vi "Motion Control.vi"(8 "error in (no error)":errorcluster) -> (0 "error out":errorcluster)   [LabVIEW 2020, in "Motion.lvlib"]
doc: "Message loop for handling messages pertaining to the acquisition of data from the hardware."
uses:
  Motion.lvlib
  support/PCT FGV CMD.ctl
  Acquisition State.ctl
  AM Configuration.ctl
  support/Message Queue/Message Cluster.ctl
  support/Message Queue/Enqueue Message (Single).vi
  support/Message Queue/Message Queue.lvlib
  <vilib>/ErrorRing/Error Ring.xnode
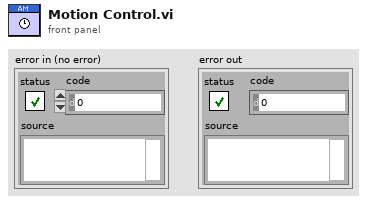
[diagram p1: front panel]
types:
  T1 = typedef "PCT FGV CMD.ctl" = enum16{"INIT", "GET", "SET"}
  T2 = typedef "Message Queue.lvlib/All Message Queues.ctl" = cluster{"UI":refnum<queue>, "Logging":refnum<queue>, "LOG":refnum<queue>, "ALARM":refnum<queue>, "Test":refnum<queue>, "Answer":refnum<queue>, "PLC":refnum<queue>, "DB":refnum<queue>, "Report":refnum<queue>, "OPC":refnum<queue>, "Procedure":refnum<queue>, "PalmSens":refnum<queue>, "SYS 7000 Reader":refnum<queue>, "SWITCH":refnum<queue>, "MOTOR":refnum<queue>, "MOTION":refnum<queue>, "HIDEN":refnum<queue>, "VALVE":refnum<queue>, "MFC":refnum<queue>, "PUMP IN":refnum<queue>, "PUMP OUT":refnum<queue>}
  T3 = typedef "PCT Data REFs.ctl" = cluster{"PLC AI Notifier":refnum<notifier>, "PS Data Queue":refnum<queue>, "BTN Queue":refnum<queue>, "PLC DI notifier":refnum<notifier>, "Timer notifier":refnum<notifier>, "DMM PS":refnum<notifier>, "DMM Gages":refnum<notifier>, "XYZ notifier":refnum<notifier>, "Test Notifier":refnum<notifier>, "Scanner notifier":refnum<notifier>, "OPC Notifier":refnum<notifier>, "HIDEN queue":refnum<queue>}
  T4 = typedef "Motion.lvlib/AM Configuration.ctl" = cluster{"Wait":dbl, "Next Step":string, "Writer Queue":refnum<queue>, "Reset":bool, "Target":dbl[]}
  T5 = typedef "Motion.lvlib/Acquisition State.ctl" = enum16{"Idle", "Initialized"}
  T6 = cluster{"Axis":enum16{"X", "Y", "Z", "A"}, "dValue":dbl}
  T7 = cluster{"Type CMD":string, "Mode CMD":string, "Main CMD":string}
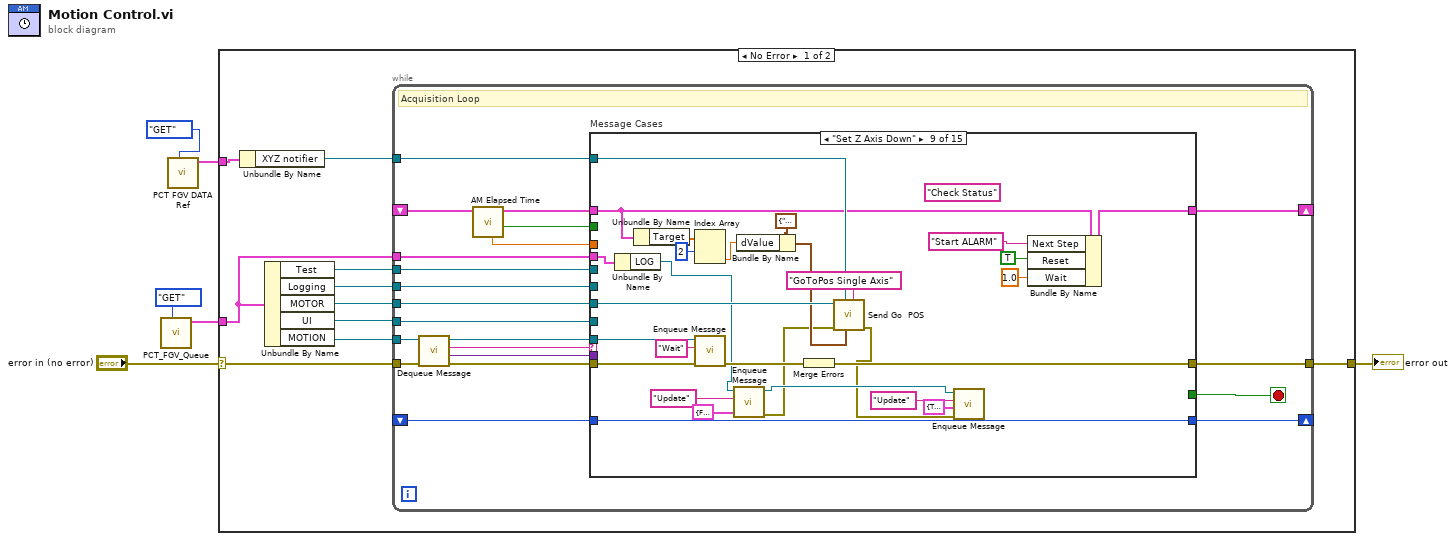
[diagram p0: block diagram]
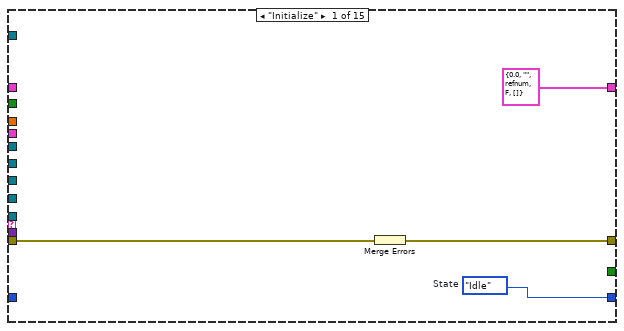
[diagram p2: hidden frame]
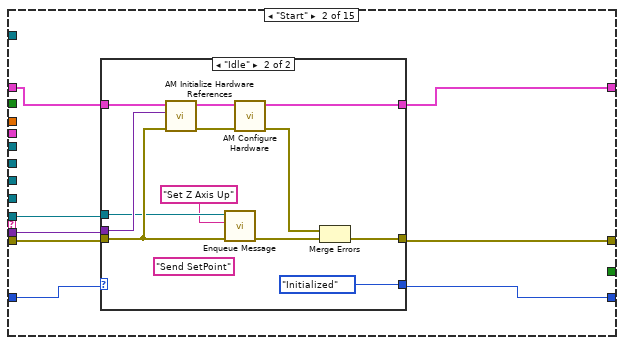
[diagram p3: hidden frame]
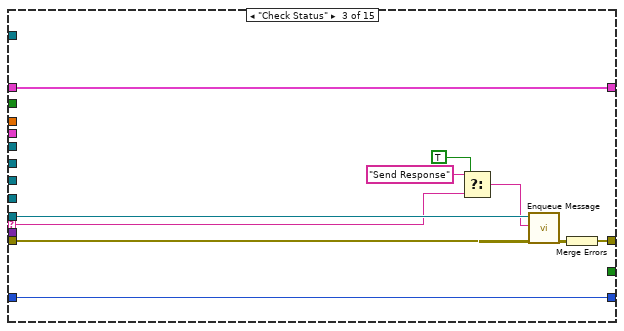
[diagram p5: hidden frame]
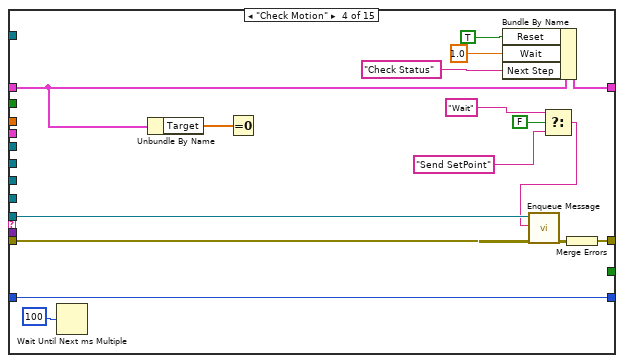
[diagram p6: hidden frame]
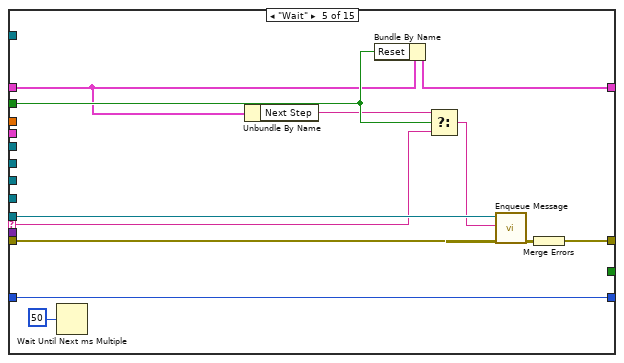
[diagram p7: hidden frame]
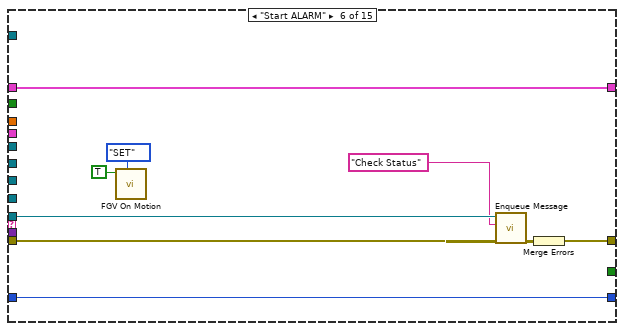
[diagram p8: hidden frame]
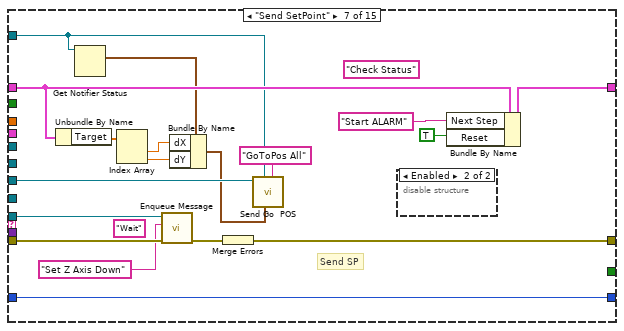
[diagram p9: hidden frame]
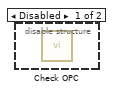
[diagram p10: hidden frame]
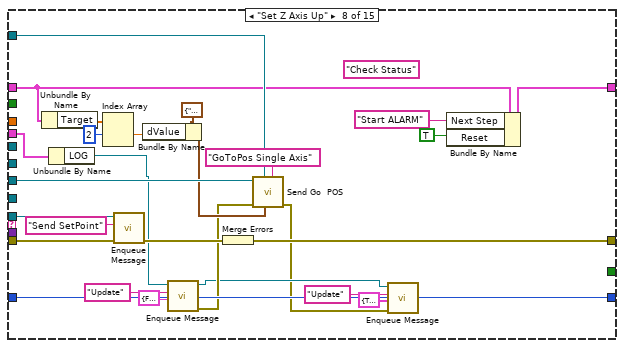
[diagram p11: hidden frame]
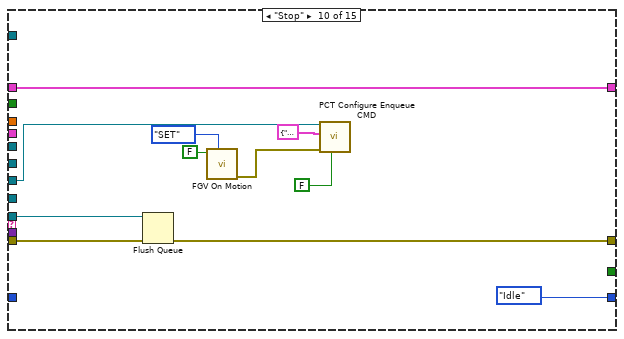
[diagram p12: hidden frame]
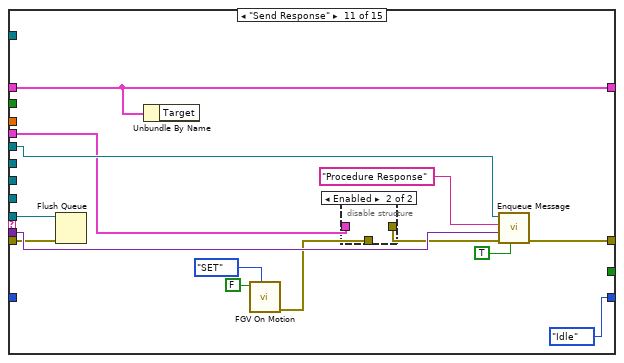
[diagram p13: hidden frame]
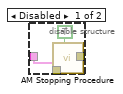
[diagram p14: hidden frame]
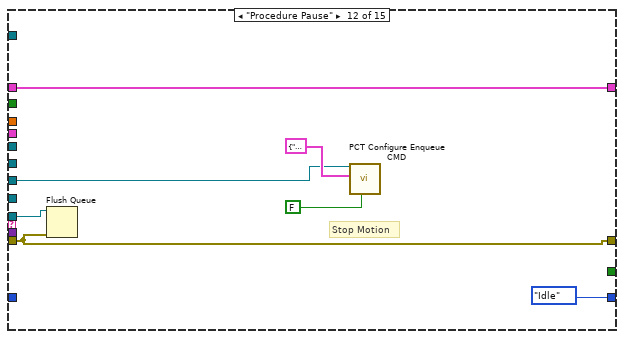
[diagram p15: hidden frame]
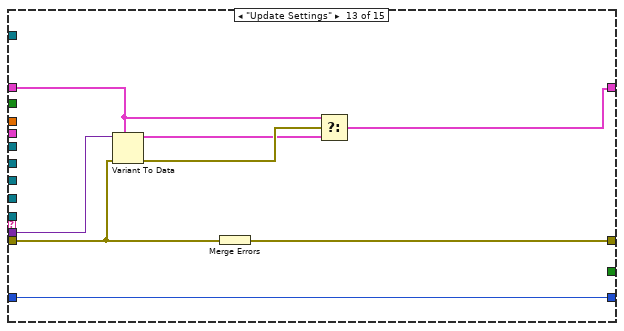
[diagram p16: hidden frame]
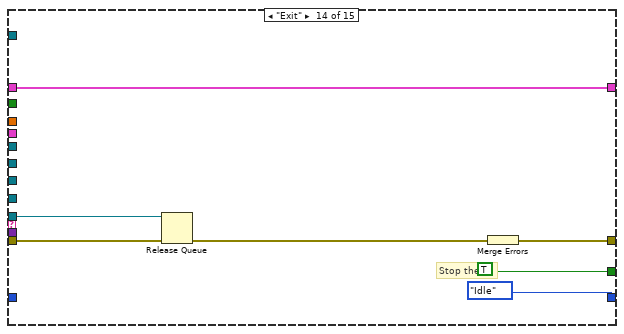
[diagram p17: hidden frame]
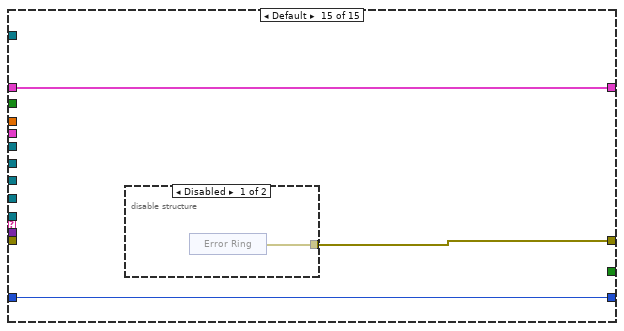
[diagram p18: hidden frame]
diagram:
  n1 = call "PCT_FGV_Queue.vi"("CMD"=PCT_FGV_CMD."GET") -> ("Message Queues out"=w4:T2)  [unwired: 9 in, 1 out]
  n2 = call "PCT FGV DATA Ref.vi"("CMD"=PCT_FGV_CMD."GET") -> ("Data REF"=w2:T3)  [unwired: 9 in, 1 out]
  n3 = case shown="No Error" "error in (no error)" {
    selector: "error in (no error)" -> [w14 w241]
    tunnel: w4 -> [w12 _]
    tunnel: [w15 w241] -> w6
    tunnel: w2 -> [w10 _]
    frame No Error {
      n4 = Unbundle By Name(w10) -> ("XYZ notifier"=w7:refnum<notifier>)
      n5 = Unbundle By Name(w12) -> ("Test"=w9:refnum<queue>, "Logging"=w8:refnum<queue>, "MOTOR"=w11:refnum<queue>, "UI"=w13:refnum<queue>, "MOTION"=w16:refnum<queue>)
      n6 = while {
        tunnel: w16 -> [w31]
        shift-right: [w37] -> _
        shift-left: _ -> [w20]
        tunnel: w13 -> [w27]
        shift-right: [w29] -> _
        shift-left: _ -> [w30]
        tunnel: w12 -> [w23]
        tunnel: w14 -> [w35]
        tunnel: [w21] -> w15
        tunnel: w11 -> [w22]
        tunnel: w9 -> [w19]
        tunnel: w8 -> [w18]
        tunnel: w7 -> [w17]
        stop <- w36 stop-if-true
        # "Acquisition Loop"
        n7 = call "Dequeue Message.vi"("error in (no error)"=w35, "Message Queue"=w31) -> ("error out"=w34:errorcluster, "Message Data"=w32:variant, "Message"=w33:string, "dup Message Queue"=w28:refnum<queue>)  [unwired: 6 in]
        n8 = call "AM Elapsed Time.vi"("AM Refs in"=w20) -> ("Time has Elapsed"=w25:bool, "AM Refs out"=w26:T4, "Elapsed Time (s)"=w24:dbl)  [unwired: 8 in]
        n9 = case "Message Cases" shown="\"Set Z Axis Down\"" w33 {
          selector: w33 -> [_ _ w68 _ w94 _ _ _ _ _ _ _ _ _ _]
          tunnel: w28 -> [_ w46 w70 w86 w98 w107 w125 w152 w180 w194 w206 w218 _ w230 _]
          tunnel: w34 -> [w40 w47 w71 w87 w99 w108 w126 w153 w181 w192 w202 w217 w222 w232 _]
          tunnel: [w41 w49 w73 w89 w101 w110 w128 w155 w183 w191 w200 w217 w228 w234 w236] -> w21
          tunnel: w26 -> [_ w48 w66 w77 w92 w106 w124 w142 w169 w195 w204 w220 w224 w233 w238]
          tunnel: [T4 {"Wait"=0.0, "Next Step"="", "Writer Queue"=refnum, "Reset"=FALSE, "Target"=[]} ("Data Cluster") w45 w66 w82 w95 w106 w123 w151 w179 w195 w204 w220 w223 w233 w238] -> w37
          tunnel: [_ _ _ _ _ _ _ _ _ _ _ _ _ TRUE _] -> w36
          tunnel: w32 -> [_ w42 _ _ _ _ _ _ _ _ w208 _ w227 _ _]
          tunnel: w27 -> [_ _ _ _ _ _ _ _ _ _ _ _ _ _ _]
          tunnel: w30 -> [_ w43 w74 w90 w102 w111 w129 w156 w184 _ _ _ w221 _ w237]
          tunnel: [w39 w44 w74 w90 w102 w111 w129 w156 w184 Acquisition_State."Idle" ("Acquisition State") Acquisition_State."Idle" ("Acquisition State") Acquisition_State."Idle" ("Acquisition State") w221 Acquisition_State."Idle" ("Acquisition State") w237] -> w29
          tunnel: w25 -> [_ _ _ _ w93 _ _ _ _ _ _ _ _ _ _]
          tunnel: w24 -> [_ _ _ _ _ _ _ _ _ _ _ _ _ _ _]
          tunnel: w23 -> [_ _ _ _ _ _ _ w137 w161 _ w203 _ _ _ _]
          tunnel: w22 -> [_ _ _ _ _ _ w120 w148 w176 w189 _ w215 _ _ _]
          tunnel: w19 -> [_ _ _ _ _ _ _ _ _ _ w205 _ _ _ _]
          tunnel: w18 -> [_ _ _ _ _ _ _ _ _ _ _ _ _ _ _]
          tunnel: w17 -> [_ _ _ _ _ _ w115 w147 w175 _ _ _ _ _ _]
          frame "Initialize" {
            w39 = Acquisition_State."Idle"  # State
            # "Initialize  - Initialize is currently a no-op.  The hardware initialization takes place in the 'Start' message."
            n10 = Merge Errors(w40) -> (w41:errorcluster)
          }
          frame "Start" {
            # "Start - Configure and start the acquisition."
            n11 = case shown="\"Idle\"" w43 {
              selector: w43 -> [w50 _]
              tunnel: [w51 w64] -> w49
              tunnel: w48 -> [w52 w63]
              tunnel: w47 -> [w51 w56]
              tunnel: w46 -> [_ w54]
              tunnel: [w52 w59] -> w45
              tunnel: [w50 Acquisition_State."Initialized" ("Acquisition State")] -> w44
              tunnel: w42 -> [_ w57]
              frame "Initialized" {
                # "The system is already acquiring. Ignore the \"Start\" message."
              }
              frame "Idle" {
                (unwired) "Send SetPoint" ("Message")
                # "If the system is idle, start the acquisition."
                n12 = call "AM Initialize Hardware References.vi"("error in (no error)"=w56, "Message Data"=w57, "Hardware Resources in"=w63) -> ("error out"=w62:errorcluster, "Hardware Resources out"=w60:T4)  [unwired: 7 in]
                n13 = call-poly "Enqueue Message.vi"("error in (no error)"=w56, "Message"="Set Z Axis Up", "Message Queue"=w54) -> ("error out"=w55:errorcluster)  [unwired: 7 in, 1 out]
                n14 = call "AM Configure Hardware.vi"("error in (no error)"=w62, "Hardware Resources in"=w60) -> ("error out"=w61:errorcluster, "Hardware Resources out"=w59:T4)  [unwired: 8 in]
                n15 = Merge Errors(w61, w55) -> (w64:errorcluster)
              }
            }
          }
          frame "Check Status" {
            # "Start - Configure and start the acquisition."
            n16 = Select(t="Send Response" ("Next Step"), s=TRUE, f=w68) -> (s? t:f=w69:string)
            n17 = call-poly "Enqueue Message.vi"("error in (no error)"=w71, "Message"=w69, "Message Queue"=w70) -> ("error out"=w72:errorcluster)  [unwired: 7 in, 1 out]
            n18 = Merge Errors(w72) -> (w73:errorcluster)
          }
          frame "Check Motion" {
            # "Start - Configure and start the acquisition."
            n19 = Wait Until Next ms Multiple(millisecond multiple=u32 100) -> ()  [unwired: 1 out]
            n20 = Unbundle By Name(w77) -> ("Target"=w76:dbl[])
            n21 = Equal To 0?(x=w76) -> ()  [unwired: 1 out]
            n22 = Bundle By Name(cluster=w77, "Reset"=TRUE, "Wait"=1.0, "Next Step"="Check Status") -> (w82:T4)
            n23 = Select(t="Wait" ("Message"), s=FALSE, f="Send SetPoint" ("Message")) -> (s? t:f=w85:string)
            n24 = call-poly "Enqueue Message.vi"("error in (no error)"=w87, "Message"=w85, "Message Queue"=w86) -> ("error out"=w88:errorcluster)  [unwired: 7 in, 1 out]
            n25 = Merge Errors(w88) -> (w89:errorcluster)
          }
          frame "Wait" {
            # "Start - Configure and start the acquisition."
            n26 = Wait Until Next ms Multiple(millisecond multiple=u32 50) -> ()  [unwired: 1 out]
            n27 = Unbundle By Name(w92) -> ("Next Step"=w91:string)
            n28 = Bundle By Name(cluster=w92, "Reset"=w93) -> (w95:T4)
            n29 = Select(t=w91, s=w93, f=w94) -> (s? t:f=w97:string)
            n30 = call-poly "Enqueue Message.vi"("error in (no error)"=w99, "Message"=w97, "Message Queue"=w98) -> ("error out"=w100:errorcluster)  [unwired: 7 in, 1 out]
            n31 = Merge Errors(w100) -> (w101:errorcluster)
          }
          frame "Start ALARM" {
            # "Start - Configure and start the acquisition."
            n32 = call "FGV On Motion.vi"("CMD"=PCT_FGV_CMD."SET", "input"=TRUE) -> ()  [unwired: 8 in, 2 out]
            n33 = call-poly "Enqueue Message.vi"("error in (no error)"=w108, "Message"="Check Status" ("Next Step"), "Message Queue"=w107) -> ("error out"=w109:errorcluster)  [unwired: 7 in, 1 out]
            n34 = Merge Errors(w109) -> (w110:errorcluster)
          }
          frame "Send SetPoint" {
            (unwired) "Check Status" ("Next Step")
            (unwired) "Wait" ("Next Step")
            # "Send SP"
            # "Start - Configure and start the acquisition."
            n35 = Unbundle By Name(w124) -> ("Target"=w119:dbl[])
            n36 = Get Notifier Status(notifier=w115) -> (current notification=w114:cluster{"dX":dbl, "dY":dbl, "dZ":dbl, "dA":dbl})  [unwired: 1 in, 4 out]
            n37 = Index Array(array=w119) -> (element #1=w118:dbl, element #2=w117:dbl)  [unwired: 2 in]
            n38 = call-poly "Enqueue Message.vi"("error in (no error)"=w126, "Message"="Set Z Axis Down" ("Next Step"), "Message Queue"=w125) -> ("error out"=w127:errorcluster)  [unwired: 7 in, 1 out]
            n39 = Bundle By Name(cluster=w114, "dX"=w118, "dY"=w117) -> (w116:cluster{"dX":dbl, "dY":dbl, "dZ":dbl, "dA":dbl})
            n40 = Merge Errors(w127) -> (w128:errorcluster)
            n41 = call "Send Go  POS.vi"("Type CMD"="GoToPos All", "Parameter Data"=w116, "XYZ notifier"=w115, "Motor Queue in"=w120) -> ()  [unwired: 6 in, 2 out]
            n42 = disable-structure shown="Enabled" {
              frame Disabled {
                n43 = call "Check OPC.vi"() -> ()  [unwired: 11 in, 1 out]
              }
              frame Enabled {
              }
            }
            n44 = Bundle By Name(cluster=w124, "Next Step"="Start ALARM", "Reset"=TRUE) -> (w123:T4)
          }
          frame "Set Z Axis Up" {
            (unwired) "Check Status" ("Next Step")
            # "Start - Configure and start the acquisition."
            n45 = Unbundle By Name(w142) -> ("Target"=w144:dbl[])
            n46 = Unbundle By Name(w137) -> ("LOG"=w136:refnum<queue>)
            n47 = Index Array(array=w144, index #1=2 ("index")) -> (element #1=w143:dbl)  [unwired: 1 in, 1 out]
            n48 = call-poly "Enqueue Message.vi"("error in (no error)"=w153, "Message"="Send SetPoint", "Message Queue"=w152) -> ("error out"=w154:errorcluster)  [unwired: 7 in, 1 out]
            n49 = Bundle By Name(cluster=T6 {"Axis"=enum."Z", "dValue"=0.0}, "dValue"=w143) -> (w139:T6)
            n50 = call-poly "Enqueue Message.vi"("Message Data"=cluster{"Replace":bool, "String":string} {"Replace"=FALSE, "String"="Movement to Z Up Position: Start"}, "Message"="Update" ("Main CMD"), "Message Queue"=w136) -> ("error out"=w134:errorcluster, "dup Message Queue"=w131:refnum<queue>)  [unwired: 7 in]
            n51 = Merge Errors(w154) -> (w155:errorcluster)
            n52 = call "Send Go  POS.vi"("Type CMD"="GoToPos Single Axis", "Parameter Data"=w139, "XYZ notifier"=w147, "error in (no error)"=w134, "Motor Queue in"=w148) -> ("error out"=w130:errorcluster)  [unwired: 5 in, 1 out]
            n53 = call-poly "Enqueue Message.vi"("error in (no error)"=w130, "Message Data"=cluster{"Replace":bool, "String":string} {"Replace"=TRUE, "String"="Movement to Z Up Position: DONE"}, "Message"="Update" ("Main CMD"), "Message Queue"=w131) -> ()  [unwired: 6 in, 2 out]
            n54 = Bundle By Name(cluster=w142, "Next Step"="Start ALARM", "Reset"=TRUE) -> (w151:T4)
          }
          frame "Set Z Axis Down" {
            (unwired) "Check Status" ("Next Step")
            # "Start - Configure and start the acquisition."
            n55 = Unbundle By Name(w161) -> ("LOG"=w160:refnum<queue>)
            n56 = Unbundle By Name(w169) -> ("Target"=w172:dbl[])
            n57 = Index Array(array=w172, index #1=2 ("index")) -> (element #2=w168:dbl)  [unwired: 1 in, 1 out]
            n58 = call-poly "Enqueue Message.vi"("error in (no error)"=w181, "Message"="Wait", "Message Queue"=w180) -> ("error out"=w182:errorcluster)  [unwired: 7 in, 1 out]
            n59 = call-poly "Enqueue Message.vi"("Message Data"=cluster{"Replace":bool, "String":string} {"Replace"=FALSE, "String"="Movement to Z DownPosition: Start"}, "Message"="Update" ("Main CMD"), "Message Queue"=w160) -> ("error out"=w159:errorcluster, "dup Message Queue"=w162:refnum<queue>)  [unwired: 7 in]
            n60 = Bundle By Name(cluster=T6 {"Axis"=enum."Z", "dValue"=0.0}, "dValue"=w168) -> (w167:T6)
            n61 = Merge Errors(w182) -> (w183:errorcluster)
            n62 = call "Send Go  POS.vi"("Type CMD"="GoToPos Single Axis", "Parameter Data"=w167, "XYZ notifier"=w175, "error in (no error)"=w159, "Motor Queue in"=w176) -> ("error out"=w158:errorcluster)  [unwired: 5 in, 1 out]
            n63 = call-poly "Enqueue Message.vi"("error in (no error)"=w158, "Message Data"=cluster{"Replace":bool, "String":string} {"Replace"=TRUE, "String"="Movement to Z Down Position: DONE"}, "Message"="Update" ("Main CMD"), "Message Queue"=w162) -> ()  [unwired: 6 in, 2 out]
            n64 = Bundle By Name(cluster=w169, "Next Step"="Start ALARM", "Reset"=TRUE, "Wait"=1.0) -> (w179:T4)
          }
          frame "Stop" {
            # "Start - Configure and start the acquisition."
            n65 = Flush Queue(queue=w194, error in (no error)=w192) -> (error out=w191:errorcluster)  [unwired: 2 out]
            n66 = call "FGV On Motion.vi"("CMD"=PCT_FGV_CMD."SET", "input"=FALSE) -> ("error out"=w185:errorcluster)  [unwired: 8 in, 1 out]
            n67 = call "PCT Configure Enqueue CMD.vi"("Parameter Data"=FALSE, "error in (no error)"=w185, "CMD"=T7 {"Type CMD"="Start", "Mode CMD"="", "Main CMD"="Action-Status"}, "CMD Queue in"=w189) -> ()  [unwired: 5 in, 3 out]
          }
          frame "Send Response" {
            # "Acquire - Acquire data from the hardware. Since this is a continuous acquisition, this message will always message itself to run again."
            n68 = Flush Queue(queue=w206, error in (no error)=w202) -> ()  [unwired: 3 out]
            n69 = Unbundle By Name(w204) -> ()  [unwired: 1 out]
            n70 = call "FGV On Motion.vi"("CMD"=PCT_FGV_CMD."SET", "input"=FALSE) -> ("error out"=w196:errorcluster)  [unwired: 8 in, 1 out]
            n71 = disable-structure shown="Enabled" {
              disable-tunnel: w203 -> [w213 _]
              disable-tunnel: [w212 _] -> w201
              disable-tunnel: w196 -> [w211 _]
              frame Disabled {
                n72 = call "AM Stopping Procedure.vi"("Stop"=TRUE, "error in (no error)"=w211, "Message Queues in"=w213) -> ("error out"=w212:errorcluster)  [unwired: 8 in]
              }
              frame Enabled {
              }
            }
            n73 = call-poly "Enqueue Message.vi"("Priority Message? (F)"=TRUE, "error in (no error)"=w201, "Message Data"=w208, "Message"="Procedure Response", "Message Queue"=w205) -> ("error out"=w200:errorcluster)  [unwired: 5 in, 1 out]
          }
          frame "Procedure Pause" {
            # "Stop Motion"
            # "Acquire - Acquire data from the hardware. Since this is a continuous acquisition, this message will always message itself to run again."
            n74 = Flush Queue(queue=w218, error in (no error)=w217) -> ()  [unwired: 3 out]
            n75 = call "PCT Configure Enqueue CMD.vi"("Parameter Data"=FALSE, "CMD"=T7 {"Type CMD"="Start", "Mode CMD"="", "Main CMD"="Action-Status"}, "CMD Queue in"=w215) -> ()  [unwired: 6 in, 3 out]
          }
          frame "Update Settings" {
            # "New settings are available, update the current ones stored in the shift register with the settings sent as part of the message"
            n76 = Variant To Data(error in=w222, type=w224, Variant=w227) -> (data=w225:T4, error out=w226:errorcluster)
            n77 = Merge Errors(w222) -> (w228:errorcluster)
            n78 = Select(t=w224, s=w226, f=w225) -> (s? t:f=w223:T4)
          }
          frame "Exit" {
            # "Stop the VI"
            # "Exit - Send the Exit message to the UI Message Handler."
            n79 = Release Queue(queue=w230, error in (no error)=w232) -> (error out=w231:errorcluster)  [unwired: 1 in, 2 out]
            n80 = Merge Errors(w231) -> (w234:errorcluster)
          }
          frame Default {
            # "'Default' case only runs if there is a message that isn't defined in any of the other cases.  Output a programming error."
            n81 = disable-structure shown="Disabled" {
              disable-tunnel: [w239 _] -> w236
              frame Disabled {
                n82 = xnode "Error Ring"() -> ("error out"=w239:errorcluster)
              }
              frame Enabled {
              }
            }
          }
        }
      }
    }
    frame Error {
    }
  }
  "error out" <- w6
